vi "Rename And Move Entire Library By Path.vi"(8 "error in (no error)":errorcluster, 9 "Delete old directory if empty after move? (T)":bool=TRUE, 10 "New library path":path, 11 "Library ref in":refnum<vi>) -> (0 "error out":errorcluster, 3 "Library ref out":refnum<vi>)   [LabVIEW 2017, in "Edit LVLibs.lvlib"]
doc: "Given a new path for this library (any LabVIEW library file extension), this VI will move that VI to the new location and change its name to the new given name. Then all the member VIs and sublibraries of the library will also be moved to the new directory maintaining their relative positions. Any member of the library that was not in the same directory as the library or a sublibrary will not be moved at all. By default, the old directory will be deleted after the move if it is empty of all files. The library and all members of the library will be saved at the end of this move to ensure that all files stay in sync with each other. Other files in memory that reference the library or its members will be modified to point to the new location but will not be saved."
uses:
  <vilib>/Utility/EditLVLibs/Edit LVLibs.lvlib
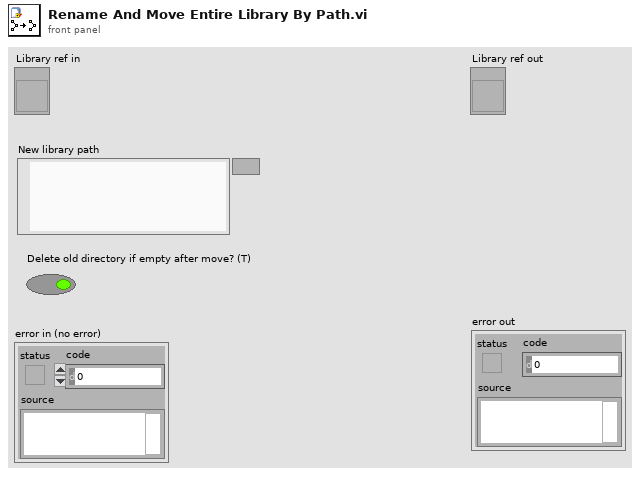
[diagram p1: front panel]
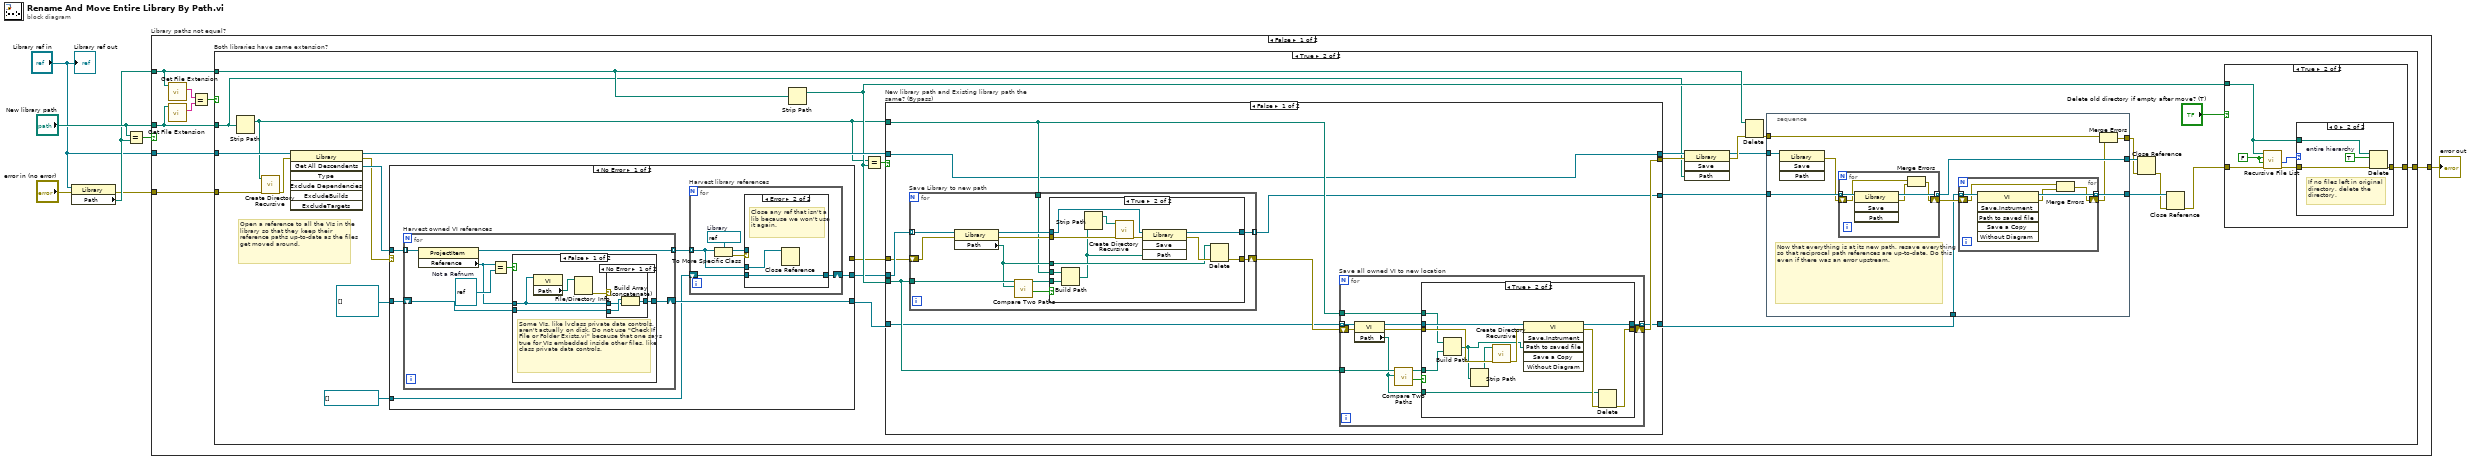
[diagram p0: block diagram]
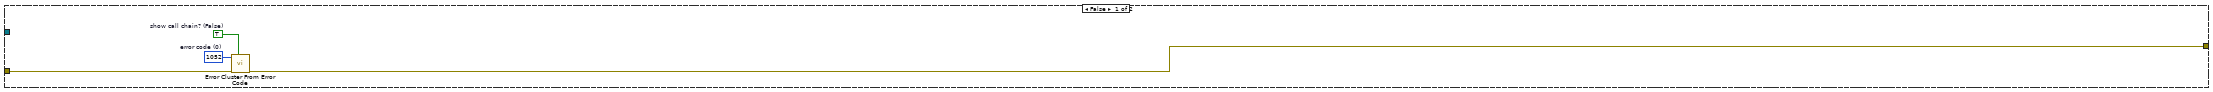
[diagram p2: hidden frame]
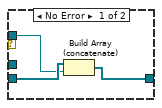
[diagram p3: hidden frame]
diagram:
  n1 = property class="Library"(reference="Library ref in", error in="error in (no error)") -> (error out=w2:errorcluster, "Path"=w4:path)  [unwired: 1 out]
  n2 = Equal?(x="New library path", y=w4) -> (x = y?=w5:bool)
  n3 = case "Library paths not equal?" shown="False" w5 {
    tunnel: [w15 w181] -> w7
    tunnel: "New library path" -> [w12 _]
    tunnel: w2 -> [w13 w181]
    tunnel: "Library ref in" -> [w14 _]
    tunnel: w4 -> [w11 _]
    frame False {
      n4 = call <vilib>:"Get File Extension.vi"("file"=w11) -> ("lowercase file extension"=w9:string)  [unwired: 6 in, 4 out]
      n5 = call <vilib>:"Get File Extension.vi"("file"=w12) -> ("lowercase file extension"=w10:string)  [unwired: 6 in, 4 out]
      n6 = Equal?(x=w9, y=w10) -> (x = y?=w8:bool)
      n7 = case "Both libraries have same extension?" shown="True" w8 {
        tunnel: [w18 w49] -> w15
        tunnel: w14 -> [_ w44]
        tunnel: w13 -> [w19 w43]
        tunnel: w12 -> [_ w21]
        tunnel: w11 -> [_ w40]
        frame False {
          w16 = TRUE  # show call chain? (False)
          w17 = 1052  # error code (0)
          n8 = call <vilib>:"Error Cluster From Error Code.vi"("show call chain? (False)"=w16, "error in (no error)"=w19, "error code (0)"=w17) -> ("error out"=w18:errorcluster)  [unwired: 6 in]
        }
        frame True {
          # "Open a reference to all the VIs in the library so that they keep their reference paths up-to-date as the files get moved around."
          n9 = Strip Path(path=w21) -> (stripped path=w20:path)  [unwired: 1 out]
          n10 = call <vilib>:"Create Directory Recursive.vi"("error in (no error)"=w43, "directory"=w20) -> ("error out"=w48:errorcluster)  [unwired: 3 in, 2 out]
          n11 = invoke class="Library" method="Get All Descendents"(reference=w44, error in=w48) -> (reference out=w37:refnum<vi>, error out=w29:errorcluster, "All Descendents"=w34:refnum<vi>[])  [unwired: 5 in, 4 out]
          n12 = case shown="No Error" w29 {
            selector: w29 -> [_ w106]
            tunnel: w34 -> [w75 _]
            tunnel: [_ w106] -> w33
            tunnel: [w70 w104] -> w32
            tunnel: [w74 w105] -> w31
            tunnel: refnum<vi>[] [] -> [w73 w105]
            tunnel: refnum<vi>[] [] -> [w71 w104]
            frame No Error {
              n13 = for "Harvest owned VI references" {
                tunnel: w75 -> [w93] mode=indexing
                tunnel: [w92] -> w72 mode=indexing
                shift-right: [w88] -> w74
                shift-left: w73 -> [w89]
                w91 = refnum<vi> refnum  # Not a Refnum
                n14 = property class="ProjectItem"(reference=w93) -> (reference out=w92:refnum<vi>, "Reference"=w87:refnum<vi>)  [unwired: 1 in, 1 out]
                n15 = Equal?(x=w87, y=w91) -> (x = y?=w90:bool)
                n16 = case shown="False" w90 {
                  tunnel: w89 -> [w98 w103]
                  tunnel: [w97 w103] -> w88
                  tunnel: w87 -> [w96 _]
                  frame False {
                    # "Some VIs, like lvclass private data controls, aren't actually on disk. Do not use \"Check If File or Folder Exists.vi\" because that one says true for VIs embedded inside other files, like class private data controls."
                    n17 = property class="VI"(reference=w96) -> ("Path"=w95:path)  [unwired: 1 in, 2 out]
                    n18 = File/Directory Info(path=w95) -> (error out=w94:errorcluster)  [unwired: 1 in, 6 out]
                    n19 = case shown="No Error" w94 {
                      tunnel: w98 -> [w101 w102]
                      tunnel: w96 -> [w100 _]
                      tunnel: [w99 w102] -> w97
                      frame No Error {
                        n20 = Build Array (concatenate)(w101, w100) -> (w99:refnum<vi>[])
                      }
                      frame Error {
                      }
                    }
                  }
                  frame True {
                  }
                }
              }
              n21 = for "Harvest library references" {
                tunnel: w72 -> [w76] mode=indexing
                shift-right: [w77] -> w70
                shift-left: w71 -> [w78]
                w81 = refnum<vi> refnum  # Library
                n22 = To More Specific Class(target class=w81, reference=w76) -> (specific class reference=w79:refnum<vi>, error out=w80:errorcluster)  [unwired: 1 in]
                n23 = case shown="Error" w80 {
                  tunnel: w79 -> [w82 _]
                  tunnel: w78 -> [w84 w86]
                  tunnel: [w83 w86] -> w77
                  tunnel: w76 -> [_ w85]
                  frame No Error {
                    n24 = Build Array (concatenate)(w84, w82) -> (w83:refnum<vi>[])
                  }
                  frame Error {
                    # "Close any ref that isn't a lib because we won't use it again."
                    n25 = Close Reference(reference=w85) -> ()  [unwired: 1 in, 1 out]
                  }
                }
              }
            }
            frame Error {
            }
          }
          n26 = Strip Path(path=w40) -> (stripped path=w35:path)  [unwired: 1 out]
          n27 = Equal?(x=w20, y=w35) -> (x = y?=w39:bool)
          n28 = case "New library path and Existing library path the same? (Bypass)" shown="False" w39 {
            tunnel: w33 -> [w107 w168]
            tunnel: w31 -> [w111 w167]
            tunnel: [w116 w168] -> w47
            tunnel: [w115 w167] -> w27
            tunnel: [w110 w165] -> w45
            tunnel: w37 -> [w108 w166]
            tunnel: w20 -> [w113 _]
            tunnel: w35 -> [w112 _]
            tunnel: [w108 w166] -> w36
            tunnel: w32 -> [w109 w165]
            frame False {
              n29 = for "Save Library to new path" {
                tunnel: w109 -> [w117] mode=indexing
                shift-right: [w122] -> w114
                shift-left: w107 -> [w118]
                tunnel: [w123] -> w110 mode=indexing
                tunnel: w112 -> [w126]
                tunnel: w113 -> [w119]
                n30 = property class="Library"(reference=w117, error in=w118) -> (reference out=w124:refnum<vi>, error out=w127:errorcluster, "Path"=w120:path)
                n31 = call <vilib>:"Compare Two Paths.vi"("Path 2"=w120, "Path 1"=w126) -> ("Path 2 Relative to Path 1?"=w121:bool, "Relative Path from 1 to 2"=w125:path)  [unwired: 6 in, 2 out]
                n32 = case shown="True" w121 {
                  tunnel: w127 -> [w129 w140]
                  tunnel: w125 -> [_ w139]
                  tunnel: w119 -> [_ w138]
                  tunnel: w124 -> [w128 w137]
                  tunnel: [w128 w134] -> w123
                  tunnel: [w129 w133] -> w122
                  tunnel: w120 -> [_ w132]
                  frame False {
                  }
                  frame True {
                    n33 = Build Path(base path=w138, name or relative path=w139) -> (appended path=w130:path)
                    n34 = Strip Path(path=w130) -> (stripped path=w131:path)  [unwired: 1 out]
                    n35 = call <vilib>:"Create Directory Recursive.vi"("error in (no error)"=w140, "directory"=w131) -> ("error out"=w136:errorcluster)  [unwired: 3 in, 2 out]
                    n36 = invoke class="Library" method="Save"(reference=w137, error in=w136, "Path"=w130) -> (reference out=w134:refnum<vi>, error out=w135:errorcluster)  [unwired: 1 in, 2 out]
                    n37 = Delete(path (use dialog)=w132, error in=w135) -> (error out=w133:errorcluster)  [unwired: 3 in, 2 out]
                  }
                }
              }
              n38 = for "Save all owned VI to new location" {
                tunnel: w111 -> [w150] mode=indexing
                shift-right: [w146] -> w116
                shift-left: w114 -> [w149]
                tunnel: [w145] -> w115 mode=indexing
                tunnel: w112 -> [w144]
                tunnel: w113 -> [w143]
                n39 = property class="VI"(reference=w150, error in=w149) -> (reference out=w147:refnum<vi>, error out=w148:errorcluster, "Path"=w141:path)
                n40 = call <vilib>:"Compare Two Paths.vi"("Path 2"=w141, "Path 1"=w144) -> ("Path 2 Relative to Path 1?"=w142:bool, "Relative Path from 1 to 2"=w151:path)  [unwired: 6 in, 2 out]
                n41 = case shown="True" w142 {
                  tunnel: w151 -> [_ w164]
                  tunnel: w148 -> [w152 w163]
                  tunnel: w147 -> [w153 w162]
                  tunnel: [w152 w157] -> w146
                  tunnel: [w153 w160] -> w145
                  tunnel: w143 -> [_ w159]
                  tunnel: w141 -> [_ w156]
                  frame False {
                  }
                  frame True {
                    n42 = Build Path(base path=w159, name or relative path=w164) -> (appended path=w155:path)
                    n43 = Strip Path(path=w155) -> (stripped path=w154:path)  [unwired: 1 out]
                    n44 = call <vilib>:"Create Directory Recursive.vi"("error in (no error)"=w163, "directory"=w154) -> ("error out"=w161:errorcluster)  [unwired: 3 in, 2 out]
                    n45 = invoke class="VI" method="Save.Instrument"(reference=w162, error in=w161, "Path to saved file"=w155) -> (reference out=w160:refnum<vi>, error out=w158:errorcluster)  [unwired: 3 in, 4 out]
                    n46 = Delete(path (use dialog)=w156, error in=w158) -> (error out=w157:errorcluster)  [unwired: 3 in, 2 out]
                  }
                }
              }
            }
            frame True {
            }
          }
          n47 = invoke class="Library" method="Save"(reference=w36, error in=w47, "Path"=w21) -> (reference out=w25:refnum<vi>, error out=w41:errorcluster)  [unwired: 1 in, 2 out]
          n48 = Delete(path (use dialog)=w40, error in=w41) -> (error out=w24:errorcluster)  [unwired: 3 in, 2 out]
          n49 = stacked-sequence {
            tunnel: [w59] -> w46
            tunnel: w45 -> [w58]
            tunnel: [w57] -> w38
            tunnel: w27 -> [w55]
            tunnel: w25 -> [w54]
            tunnel: w24 -> [w52]
            tunnel: [w50] -> w23
            frame #0 {
              # "Now that everything is at its new path, resave everything so that reciprocal path references are up-to-date. Do this even if there was an error upstream."
              n50 = invoke class="Library" method="Save"(reference=w54) -> (error out=w53:errorcluster)  [unwired: 3 in, 3 out]
              n51 = for {
                tunnel: w58 -> [w64] mode=indexing
                tunnel: [w63] -> w57 mode=indexing
                shift-right: [w60] -> w56
                shift-left: w53 -> [w62]
                n52 = invoke class="Library" method="Save"(reference=w64) -> (reference out=w63:refnum<vi>, error out=w61:errorcluster)  [unwired: 3 in, 2 out]
                n53 = Merge Errors(w62, w61) -> (w60:errorcluster)
              }
              n54 = for {
                shift-right: [w65] -> w51
                shift-left: w56 -> [w67]
                tunnel: [w69] -> w59 mode=indexing
                tunnel: w55 -> [w68] mode=indexing
                n55 = invoke class="VI" method="Save.Instrument"(reference=w68) -> (reference out=w69:refnum<vi>, error out=w66:errorcluster)  [unwired: 5 in, 4 out]
                n56 = Merge Errors(w67, w66) -> (w65:errorcluster)
              }
              n57 = Merge Errors(w52, w51) -> (w50:errorcluster)
            }
          }
          n58 = Close Reference(reference=w38, error in (no error)=w23) -> (error out=w26:errorcluster)
          n59 = Close Reference(reference=w46, error in (no error)=w26) -> (error out=w22:errorcluster)
          n60 = case shown="True" "Delete old directory if empty after move? (T)" {
            tunnel: [w169 w175] -> w49
            tunnel: w22 -> [w169 w171]
            tunnel: w35 -> [_ w174]
            frame False {
            }
            frame True {
              w173 = FALSE ("Treat LLBs as Folders?")
              n61 = call <vilib>:"Recursive File List.vi"("error in (no error)"=w171, "Continue Recursing on Error? (F)"=w173, "Treat LLBs as Folders?"=w173, "Folder Path"=w174) -> ("error out"=w170:errorcluster, "Number of Files"=w172:i32)  [unwired: 3 in, 3 out]
              n62 = case shown="0" w172 {
                tunnel: [w176 w180] -> w175
                tunnel: w170 -> [w176 w178]
                tunnel: w174 -> [_ w177]
                frame Default {
                }
                frame 0 {
                  w179 = TRUE  # entire hierarchy
                  # "If no files left in original directory, delete the directory."
                  n63 = Delete(path (use dialog)=w177, entire hierarchy (F)=w179, error in=w178) -> (error out=w180:errorcluster)  [unwired: 2 in, 2 out]
                }
              }
            }
          }
        }
      }
    }
    frame True {
    }
  }
  "error out" <- w7
  "Library ref out" <- "Library ref in"
